vi "ni579x Verify Compatibility.vi"(0 "Register Bus":refnum<class "ni579x Register Bus v1 Host.lvclass">=refnum, 11 "Error In":errorcluster) -> (4 "Register Bus (out)":refnum<class "ni579x Register Bus v1 Host.lvclass">, 15 "Error Out":errorcluster)   [LabVIEW 2015]
uses:
  <instrlib>/ni579x/Register Bus/v1/Host/ni579x Register Bus v1 Host.lvclass
  <instrlib>/ni579x/Config/v1/Shared/Types/ni579x User Command.ctl
  <instrlib>/ni579x/Config/v1/Shared/Types/ni579x User Command ID.ctl
  <instrlib>/ni579x/Register Bus/v1/Host/Public/Register Read Request.ctl
  <instrlib>/ni579x/Config/v1/Shared/Types/ni579x Register Bus Subsystem ID.ctl
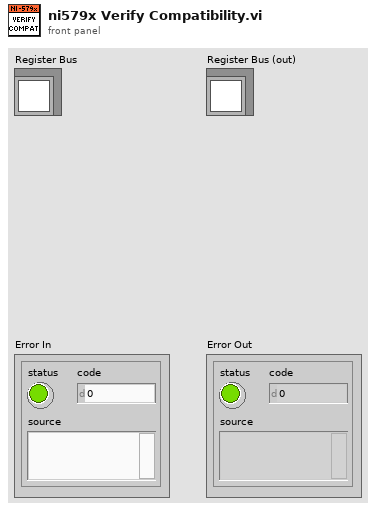
[diagram p1: front panel]
types:
  T1 = typedef "ni579x Register Bus v1 Host.lvclass/Register Read Request.ctl" = cluster{"subsystem":u8, "address":u16}
  T2 = typedef "ni579x User Command.ctl" = cluster{"User Data 0":u8, "User Data 1":u8, "User Command ID":T3}
  T3 = typedef "ni579x User Command ID.ctl" = u8
  T4 = typedef "ni579x Register Bus Subsystem ID.ctl" = u8
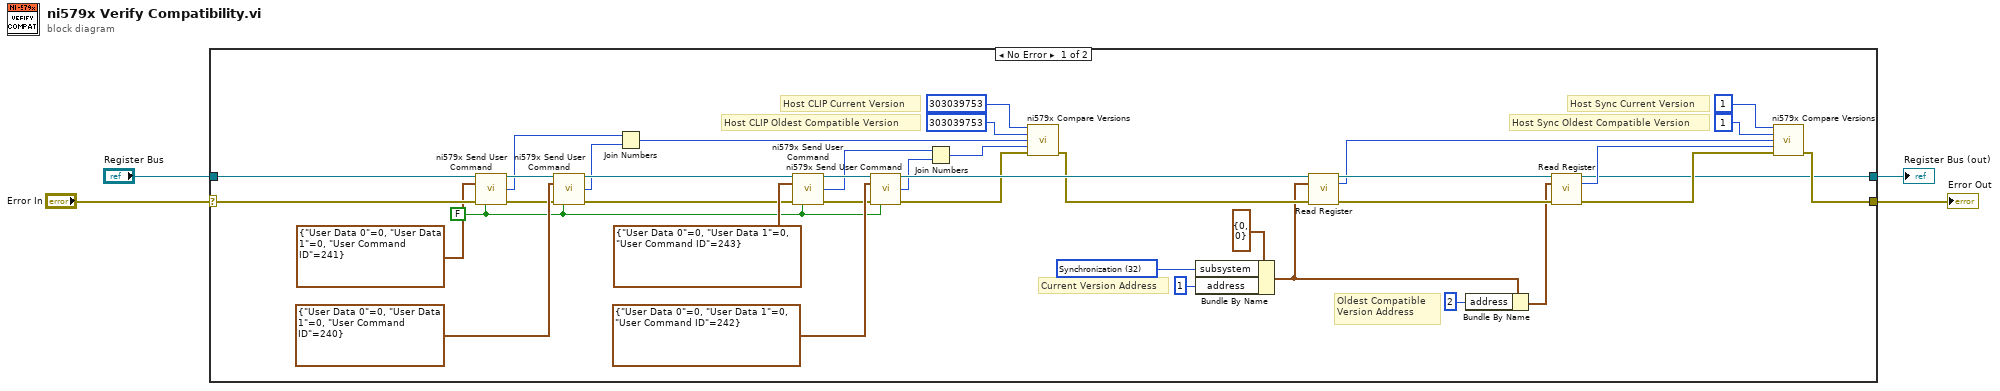
[diagram p0: block diagram]
diagram:
  n1 = case shown="No Error" "Error In" {
    selector: "Error In" -> [w42 w45]
    tunnel: [w22 w45] -> w3
    tunnel: "Register Bus" -> [w43 w44]
    tunnel: [w21 w44] -> w1
    frame No Error {
      w7 = FALSE ("wait for completion?")
      w35 = T4 32 items=["FAM Register Operation"=0, "User Command"=16, "Synchronization"=32] ("Subsystem ID")
      # "Host CLIP Oldest Compatible Version"
      # "Host CLIP Current Version"
      # "Host Sync Oldest Compatible Version"
      # "Host Sync Current Version"
      # "Oldest Compatible \nVersion Address"
      # "Current Version Address"
      n2 = call <instrlib>:"ni579x Send User Command.vi"("Register Bus"=w43, "User Command"=T2 {"User Data 0"=0, "User Data 1"=0, "User Command ID"=241}, "Error In"=w42, "wait for completion?"=w7) -> ("Register Bus (out)"=w20:refnum<class "ni579x Register Bus v1 Host.lvclass">, "user return value"=w14:u16, "Error Out"=w19:errorcluster)  [unwired: 7 in, 2 out]
      n3 = call <instrlib>:"ni579x Send User Command.vi"("Register Bus"=w20, "User Command"=T2 {"User Data 0"=0, "User Data 1"=0, "User Command ID"=240}, "Error In"=w19, "wait for completion?"=w7) -> ("Register Bus (out)"=w16:refnum<class "ni579x Register Bus v1 Host.lvclass">, "user return value"=w13:u16, "Error Out"=w15:errorcluster)  [unwired: 7 in, 2 out]
      n4 = Join Numbers(hi=w14, lo=w13) -> ((hi.lo)=w10:u32)
      n5 = call <instrlib>:"ni579x Send User Command.vi"("Register Bus"=w16, "User Command"=T2 {"User Data 0"=0, "User Data 1"=0, "User Command ID"=243}, "Error In"=w15, "wait for completion?"=w7) -> ("Register Bus (out)"=w17:refnum<class "ni579x Register Bus v1 Host.lvclass">, "user return value"=w12:u16, "Error Out"=w18:errorcluster)  [unwired: 7 in, 2 out]
      n6 = call <instrlib>:"ni579x Send User Command.vi"("Register Bus"=w17, "User Command"=T2 {"User Data 0"=0, "User Data 1"=0, "User Command ID"=242}, "Error In"=w18, "wait for completion?"=w7) -> ("Register Bus (out)"=w37:refnum<class "ni579x Register Bus v1 Host.lvclass">, "user return value"=w11:u16, "Error Out"=w8:errorcluster)  [unwired: 7 in, 2 out]
      n7 = Join Numbers(hi=w12, lo=w11) -> ((hi.lo)=w9:u32)
      n8 = call <instrlib>:"ni579x Compare Versions.vi"("Host Current Version"=u32 303039753, "Host Oldest Compatible Version"=u32 303039753 ("Host Current Version"), "FPGA Current Version"=w10, "FPGA Oldest Compatible Version"=w9, "Error In"=w8) -> ("Error Out"=w36:errorcluster)  [unwired: 10 in]
      n9 = Bundle By Name(cluster=T1 {"subsystem"=0, "address"=0} ("register read request"), "subsystem"=w35, "address"=u16 1) -> (w30:T1)
      n10 = call <instrlib>:"Read Register.vi"("session in"=w37, "register read request"=w30, "error in"=w36) -> ("session out"=w32:refnum<class "ni579x Register Bus v1 Host.lvclass">, "data"=w24:u32, "error out"=w31:errorcluster)  [unwired: 10 in]
      n11 = Bundle By Name(cluster=w30, "address"=u16 2) -> (w28:T1)
      n12 = call <instrlib>:"Read Register.vi"("session in"=w32, "register read request"=w28, "error in"=w31) -> ("session out"=w21:refnum<class "ni579x Register Bus v1 Host.lvclass">, "data"=w23:u32, "error out"=w25:errorcluster)  [unwired: 10 in]
      n13 = call <instrlib>:"ni579x Compare Versions.vi"("Host Current Version"=u32 1, "Host Oldest Compatible Version"=u32 1 ("Host Current Version"), "FPGA Current Version"=w24, "FPGA Oldest Compatible Version"=w23, "Error In"=w25) -> ("Error Out"=w22:errorcluster)  [unwired: 10 in]
    }
    frame Error {
    }
  }
  "Register Bus (out)" <- w1
  "Error Out" <- w3
